vi "计算起摆时输出电压值-子.vi"(2 "起摆系数":dbl, 3 "计算后的摆臂角度":dbl) -> (0 "是否在规定电压范围内":bool, 1 "输出电压值":dbl)   [LabVIEW 2015]
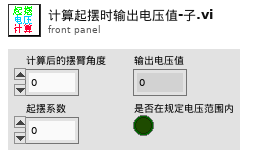
[diagram p1: front panel]
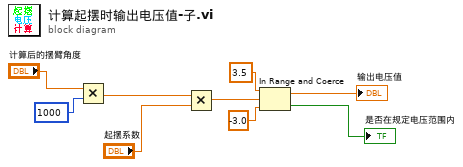
[diagram p0: block diagram]
diagram:
  n1 = Multiply(x="计算后的摆臂角度", y=1000) -> (x*y=w8:dbl)
  n2 = Multiply(x=w8, y="起摆系数") -> (x*y=w7:dbl)
  n3 = In Range and Coerce(upper limit=3.5 ("上限"), x=w7, lower limit=-3.0 ("下限")) -> (coerced(x)=→"输出电压值":dbl, In Range?=→"是否在规定电压范围内":bool)
